vi "R2050-40Operation.vi"(10 "pressure_drop (psia)":dbl=10.0, 11 "angle (deg)":dbl) -> (3 "flow (m³/s)":dbl)   [LabVIEW 2020]
doc: "Computes liquid flow through an R2050-40 valve given its opening angle."
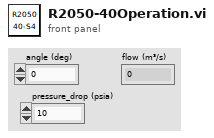
[diagram p1: front panel]
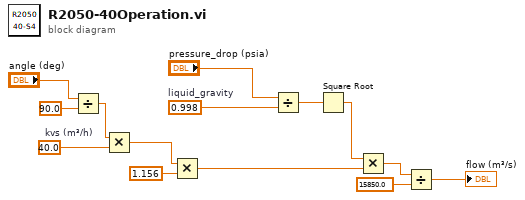
[diagram p0: block diagram]
diagram:
  w11 = 0.998  # liquid_gravity
  w7 = 40.0  # kvs (m³/h)
  n1 = Divide(x="angle (deg)", y=90.0) -> (x/y=w6:dbl)
  n2 = Multiply(x=w6, y=w7) -> (x*y=w5:dbl)
  n3 = Multiply(x=w5, y=1.156) -> (x*y=w8:dbl)
  n4 = Divide(x="pressure_drop (psia)", y=w11) -> (x/y=w10:dbl)
  n5 = Square Root(x=w10) -> (sqrt(x)=w9:dbl)
  n6 = Multiply(x=w9, y=w8) -> (x*y=w4:dbl)
  n7 = Divide(x=w4, y=15850.0) -> (x/y=→"flow (m³/s)":dbl)
